vi "Center Text.vi"(8 "error in (no error)":errorcluster, 11 "Image Gallery in":refnum<class "Image Gallery.lvclass">) -> (0 "error out":errorcluster, 3 "Image Gallery out":refnum<class "Image Gallery.lvclass">)   [LabVIEW 2012, in "ImageGallery.lvlib" / "Image Gallery.lvclass"]
uses:
  Image Gallery.lvclass
  <vilib>/Utility/miscctls.llb/LVPositionTypeDef.ctl
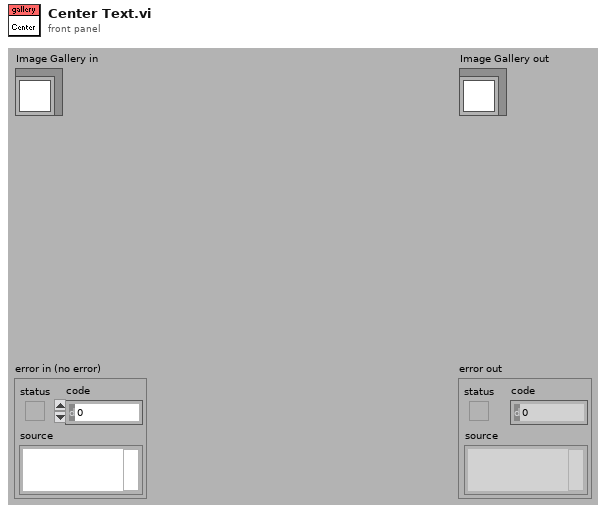
[diagram p1: front panel]
types:
  T1 = typedef "LVPositionTypeDef.ctl" = cluster{"Left":i32, "Top":i32}
  T2 = typedef "imagedata.ctl" = cluster{"image type":i32, "image depth":i32, "image":u8[], "mask":u8[], "colors":u32[], "Rectangle":cluster{"left":i16, "top":i16, "right":i16, "bottom":i16}}
  T3 = cluster{"left":i16, "top":i16, "right":i16, "bottom":i16}
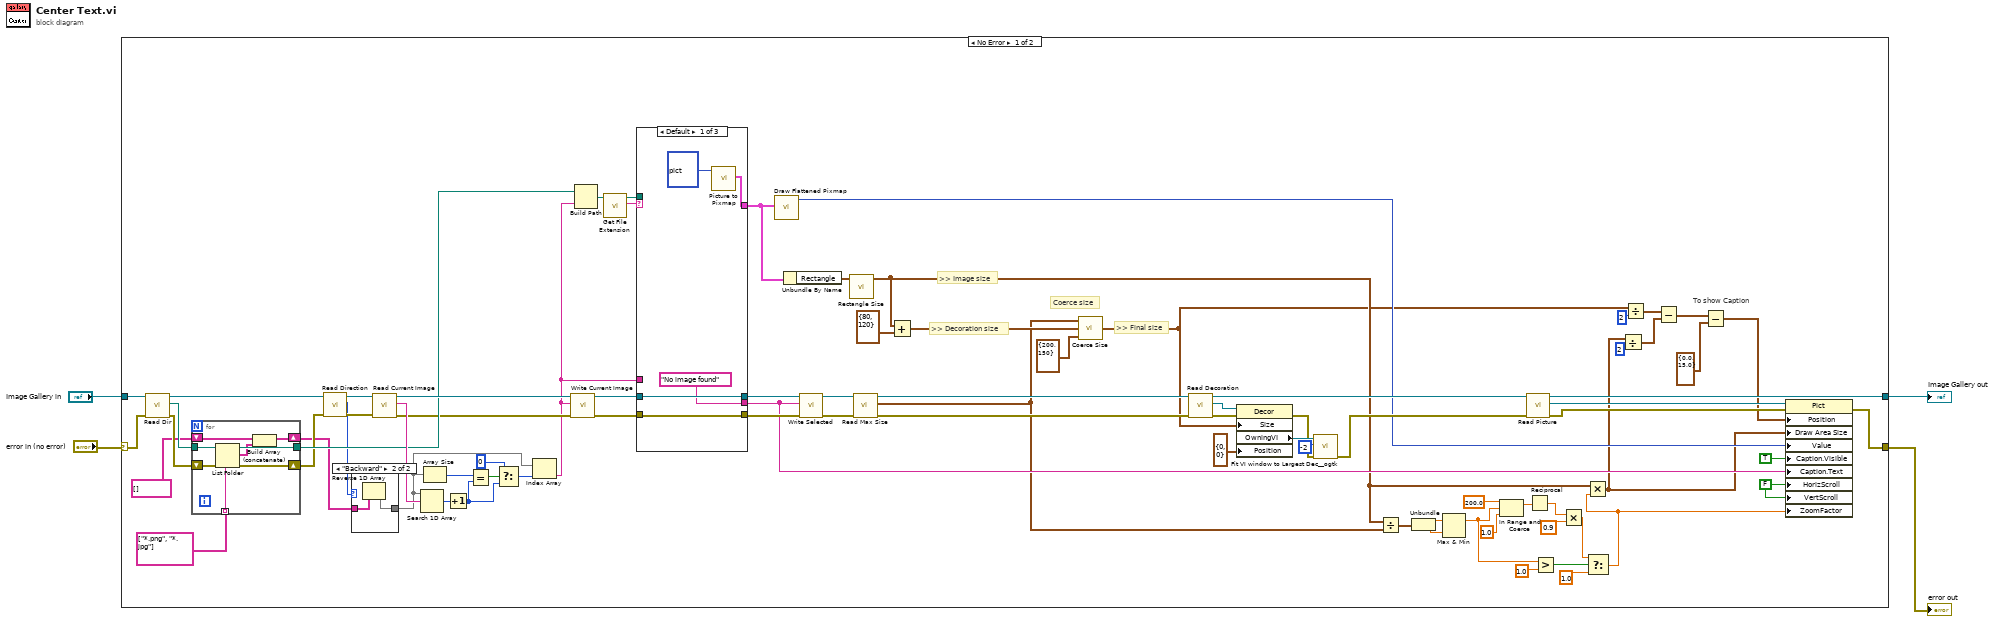
[diagram p0: block diagram]
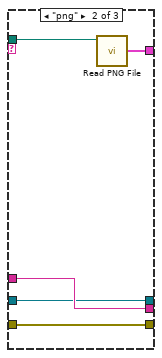
[diagram p3: hidden frame]
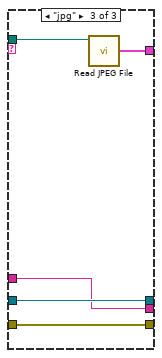
[diagram p4: hidden frame]
diagram:
  n1 = case shown="No Error" "error in (no error)" {
    selector: "error in (no error)" -> [w53 w113]
    tunnel: [w40 w113] -> w1
    tunnel: [w83 w112] -> w2
    tunnel: "Image Gallery in" -> [w54 w112]
    frame No Error {
      w17 = FALSE ("Horizontal Scrollbar Visible")
      # ">> Final size"
      # "Coerce size"
      # ">> Decoration size"
      # ">> Image size"
      # "To show Caption"
      n2 = call-dynamic "Read Dir.vi"("error in (no error)"=w53, "Image Gallery.lvclass in"=w54) -> ("error out"=w80:errorcluster, "Dir"=w81:path, "Image Gallery.lvclass out"=w52:refnum<class "Image Gallery.lvclass">)  [unwired: 7 out]
      n3 = for {
        tunnel: w81 -> [w93]
        tunnel: [w91] -> w77
        tunnel: string[] ["*.png", "*.jpg"] -> [w89] mode=indexing
        shift-right: [w90] -> w50
        shift-left: w80 -> [w92]
        shift-right: [w86] -> w20
        shift-left: string[] [] ("filenames") -> [w88]
        n4 = List Folder(path=w93, pattern=w89, error in=w92) -> (path out=w91:path, filenames=w87:string[], error out=w90:errorcluster)  [unwired: 2 out]
        n5 = Build Array (concatenate)(w88, w87) -> (w86:string[])
      }
      n6 = call-dynamic "Read Direction.vi"("error in (no error)"=w50, "Image Gallery.lvclass in"=w52) -> ("error out"=w49:errorcluster, "Direction"=w48:enum16{"Forward", "Backward"}, "Image Gallery.lvclass out"=w51:refnum<class "Image Gallery.lvclass">)  [unwired: 7 out]
      n7 = case shown="\"Backward\"" w48 {
        tunnel: w20 -> [w94 w96]
        tunnel: [w94 w95] -> w47
        frame "Forward", Default {
        }
        frame "Backward" {
          n8 = Reverse 1D Array(array=w96) -> (reversed array=w95:string[])
        }
      }
      n9 = call-dynamic "Read Current Image.vi"("error in (no error)"=w49, "Image Gallery.lvclass in"=w51) -> ("error out"=w71:errorcluster, "Current Image"=w79:string, "Image Gallery.lvclass out"=w78:refnum<class "Image Gallery.lvclass">)  [unwired: 7 out]
      n10 = Search 1D Array(1D array=w47, element=w79) -> (index of element=w60:i32)  [unwired: 1 out]
      n11 = Array Size(array=w47) -> (size(s)=w59:i32)
      n12 = Increment(x=w60) -> (x+1=w57:i32)
      n13 = Equal?(x=w59, y=w57) -> (x = y?=w58:bool)
      n14 = Select(t=0, s=w58, f=w57) -> (s? t:f=w56:i32)
      n15 = Index Array(array=w47, index=w56) -> (element=w27:string)
      n16 = call-dynamic "Write Current Image.vi"("error in (no error)"=w71, "Current Image"=w27, "Image Gallery.lvclass in"=w78) -> ("error out"=w33:errorcluster, "Image Gallery.lvclass out"=w34:refnum<class "Image Gallery.lvclass">)  [unwired: 7 out]
      n17 = Build Path(base path=w77, name or relative path=w27) -> (appended path=w76:path)
      n18 = call <vilib>:"Get File Extension.vi"("file"=w76) -> ("lowercase file extension"=w75:string, "dup file"=w74:path)  [unwired: 1 in, 8 out]
      n19 = case shown="Default" w75 {
        tunnel: w74 -> [_ w106 w111]
        tunnel: [w100 w105 w110] -> w70
        tunnel: w34 -> [w98 w103 w109]
        tunnel: w33 -> [w99 w102 w108]
        tunnel: [w99 w102 w108] -> w32
        tunnel: [w98 w103 w109] -> w31
        tunnel: ["No image found" ("pattern") w104 w107] -> w26
        tunnel: w27 -> [_ w104 w107]
        frame Default {
          n20 = call <vilib>:"Picture to Pixmap.vi"("picture"=picture bytes[51230] ("new picture 2")) -> ("image data"=w100:T2)  [unwired: 3 in, 7 out]
        }
        frame "png" {
          n21 = call <vilib>:"Read PNG File.vi"("path to PNG file"=w106) -> ("image data"=w105:T2)  [unwired: 1 in, 9 out]
        }
        frame "jpg" {
          n22 = call <vilib>:"Read JPEG File.vi"("path to JPEG file"=w111) -> ("image data"=w110:T2)  [unwired: 1 in, 9 out]
        }
      }
      n23 = call <vilib>:"Draw Flattened Pixmap.vi"("image data"=w70) -> ("new picture"=w35:picture)  [unwired: 1 in, 7 out]
      n24 = Unbundle By Name(w70) -> ("Rectangle"=w69:T3)
      n25 = call-dynamic "Write Selected.vi"("error in (no error)"=w32, "Selected"=w26, "Dialog.lvclass in"=w31) -> ("error out"=w46:errorcluster, "Dialog.lvclass out"=w44:refnum<class "Image Gallery.lvclass">)  [unwired: 7 out]
      n26 = call "Rectangle Size.vi"("Rectangle"=w69) -> ("Rect Size"=w15:cluster{"width":i32, "height":i32})  [unwired: 10 out]
      n27 = call-dynamic "Read Max Size.vi"("error in (no error)"=w46, "Dialog.lvclass in"=w44) -> ("error out"=w45:errorcluster, "Max Size"=w23:cluster{"Width":i32, "Height":i32}, "Dialog.lvclass out"=w43:refnum<class "Image Gallery.lvclass">)  [unwired: 7 out]
      n28 = Add(x=w15, y=cluster{"Width":i32, "Height":i32} {"Width"=80, "Height"=120}) -> (x+y=w25:cluster{i32, i32})
      n29 = call "Coerce Size.vi"("Min Size"=cluster{"Width":i32, "Height":i32} {"Width"=200, "Height"=150}, "Size"=w25, "Max Size"=w23) -> ("Coerced Size"=w13:cluster{"Width":i32, "Height":i32})  [unwired: 2 out]
      n30 = call-dynamic "Read Decoration.vi"("error in (no error)"=w45, "Dialog.lvclass in"=w43) -> ("error out"=w65:errorcluster, "Decoration"=w73:refnum<vi>, "Dialog.lvclass out"=w82:refnum<class "Image Gallery.lvclass">)  [unwired: 7 out]
      n31 = property class="Decor"(reference=w73, error in=w65, "Size"=w13, "Position"=T1 {"Left"=0, "Top"=0}) -> (error out=w41:errorcluster, "OwningVI"=w67:refnum<vi>)  [unwired: 1 out]
      n32 = call <userlib>:"Fit VI window to Largest Dec__ogtk.vi"("error in (no error)"=w41, "border spacing (2 px)"=-2, "VI Ref (calling VI)"=w67) -> ("error out"=w42:errorcluster)  [unwired: 4 out]
      n33 = Divide(x=w15, y=w23) -> (x/y=w30:cluster{dbl, dbl})
      n34 = Unbundle(w30) -> (w29:dbl, w28:dbl)
      n35 = Max & Min(x=w29, y=w28) -> (max(x,y)=w10:dbl)  [unwired: 1 out]
      n36 = In Range and Coerce(upper limit=200.0 ("lower limit"), x=w10, lower limit=1.0) -> (coerced(x)=w16:dbl)  [unwired: 1 out]
      n37 = call-dynamic "Read Picture.vi"("error in (no error)"=w42, "Image Gallery.lvclass in"=w82) -> ("error out"=w39:errorcluster, "Picture"=w72:refnum<vi>, "Image Gallery.lvclass out"=w83:refnum<class "Image Gallery.lvclass">)  [unwired: 7 out]
      n38 = Reciprocal(x=w16) -> (1/x=w11:dbl)
      n39 = Greater?(x=w10, y=1.0 ("lower limit")) -> (0:w8:bool)
      n40 = Multiply(x=w11, y=0.9 ("lower limit")) -> (x*y=w7:dbl)
      n41 = Select(t=w7, s=w8, f=1.0 ("lower limit")) -> (s? t:f=w5:dbl)
      n42 = Multiply(x=w15, y=w5) -> (x*y=w14:cluster{"width":dbl, "height":dbl})
      n43 = Divide(x=w14, y=2) -> (x/y=w61:cluster{"width":dbl, "height":dbl})
      n44 = Divide(x=w13, y=2) -> (x/y=w85:cluster{"Width":dbl, "Height":dbl})
      n45 = Subtract(x=w85, y=w61) -> (x-y=w38:cluster{dbl, dbl})
      n46 = Subtract(x=w38, y=cluster{dbl, dbl} {0.0, 15.0}) -> (x-y=w37:cluster{dbl, dbl})
      n47 = property class="Pict"(reference=w72, error in=w39, "Position"=w37, "Draw Area Size"=w14, "Value"=w35, "Caption.Visible"=TRUE, "Caption.Text"=w26, "HorizScroll"=w17, "VertScroll"=w17, "ZoomFactor"=w5) -> (error out=w40:errorcluster)  [unwired: 1 out]
    }
    frame Error {
    }
  }
  "error out" <- w1
  "Image Gallery out" <- w2
